vi "Main.vi"() -> ()   [LabVIEW 2014]
uses:
  <vilib>/myRIO/Common/Instrument Driver Framework/myRIO v1.0/PWM/vis/myRIO v1.1 Open PWM.vi
  <vilib>/myRIO/Common/Instrument Driver Framework/myRIO v1.0/UART/vis/myRIO v1.0 Close UART.vi
  <vilib>/myRIO/Common/Instrument Driver Framework/Utilities/vis/Validate Channels.vi
  <vilib>/myRIO/Common/Instrument Driver Framework/myRIO v1.0/PWM/vis/myRIO v1.0 Reserve PWM.vi
  <vilib>/myRIO/Common/Instrument Driver Framework/myRIO v1.0/PWM/vis/myRIO v1.0 Build MUX Configuration PWM.vi
  <vilib>/myRIO/Common/Instrument Driver Framework/myRIO v1.0/Resource Manager/vis/myRIO v1.0 Reserve Channel List.vi
  <vilib>/myRIO/Common/Instrument Driver Framework/myRIO v1.0/Resource Manager/vis/myRIO v1.0 Create Configuration List.vi
  <vilib>/myRIO/Common/Instrument Driver Framework/myRIO v1.0/Resource Manager/vis/myRIO v1.0 Reserve Channel.vi
  <vilib>/myRIO/Common/Instrument Driver Framework/myRIO v1.0/Resource Manager/vis/myRIO v1.0 Unreserve Channel.vi
  <vilib>/myRIO/Common/Instrument Driver Framework/myRIO v1.0/Resource Manager/vis/myRIO v1.0 Build Mutex Name.vi
  <vilib>/Utility/VariantDataType/GetNumericInfo.vi
  <vilib>/Utility/error.llb/Error Cluster From Error Code.vi
  <vilib>/myRIO/Common/Instrument Driver Framework/myRIO v1.0/myRIO v1.1 Open.vi
  <vilib>/myRIO/Common/Instrument Driver Framework/Utilities/vis/IO Manager.vi
  <vilib>/myRIO/Common/Instrument Driver Framework/Utilities/vis/Configuration Manager.vi
  <vilib>/myRIO/Common/Instrument Driver Framework/myRIO v1.0/Resource Manager/vis/myRIO v1.0 Configure IO.vi
  <vilib>/myRIO/Common/Instrument Driver Framework/myRIO v1.0/myRIO v1.0 Close.vi
  <vilib>/myRIO/Common/Instrument Driver Framework/myRIO v1.0/PWM/vis/myRIO v1.0 Write PWM.vi
  <vilib>/myRIO/Common/Instrument Driver Framework/Utilities/vis/FPGA Ref Manager.vi
  <vilib>/myRIO/Common/Instrument Driver Framework/myRIO v1.0/myRIO v1.0 Reset FPGA.vi
  <vilib>/myRIO/Common/Instrument Driver Framework/myRIO v1.0/IRQ/vis/myRIO v1.0 IRQ Info FGV.vi
  <vilib>/myRIO/Common/Instrument Driver Framework/myRIO v1.0/IRQ/vis/myRIO v1.0 Timer IRQ Info FGV.vi
  <vilib>/myRIO/Common/Instrument Driver Framework/myRIO v1.0/IRQ/vis/myRIO v1.0 ISR Agent.vi
  <vilib>/myRIO/Instrument Drivers/Utilities/Utilities.lvlib
  <vilib>/myRIO/Instrument Drivers/Onboard IO/PWM/PWM.lvlib
panel:
  in  "freq [Hz] 4":dbl=50.0
  in  "null offset 4":bool
  in  "position [%FS] 4":dbl(slide) scale=-200.0..200.0
  out "duty cycle [%] 4":dbl
  out "pulse width [ms] 4":dbl=1.5
  out "offset [%FS] 4":dbl
  out "pulse width [ms] 3":dbl=1.5
  out "duty cycle [%] 3":dbl
  out "offset [%FS] 3":dbl
  in  "null offset 3":bool
  in  "freq [Hz] 3":dbl=50.0
  in  "position [%FS] 3":dbl(slide) scale=-200.0..200.0
  in  "freq [Hz] 2":dbl=50.0
  in  "null offset 2":bool
  in  "position [%FS] 2":dbl(slide) scale=-200.0..200.0
  out "duty cycle [%] 2":dbl
  out "pulse width [ms] 2":dbl=1.5
  out "offset [%FS] 2":dbl
  out "duty cycle [%]":dbl
  out "pulse width [ms]":dbl=1.5
  out "offset [%FS]":dbl
  in  "freq [Hz]":dbl=50.0
  in  "null offset":bool
  in  "position [%FS]":dbl(slide) scale=-200.0..200.0
  in  "[ESC]":bool
  # "Servo  1"
  # "Servo  2"
  # "Servo  4"
  # "Servo  3"
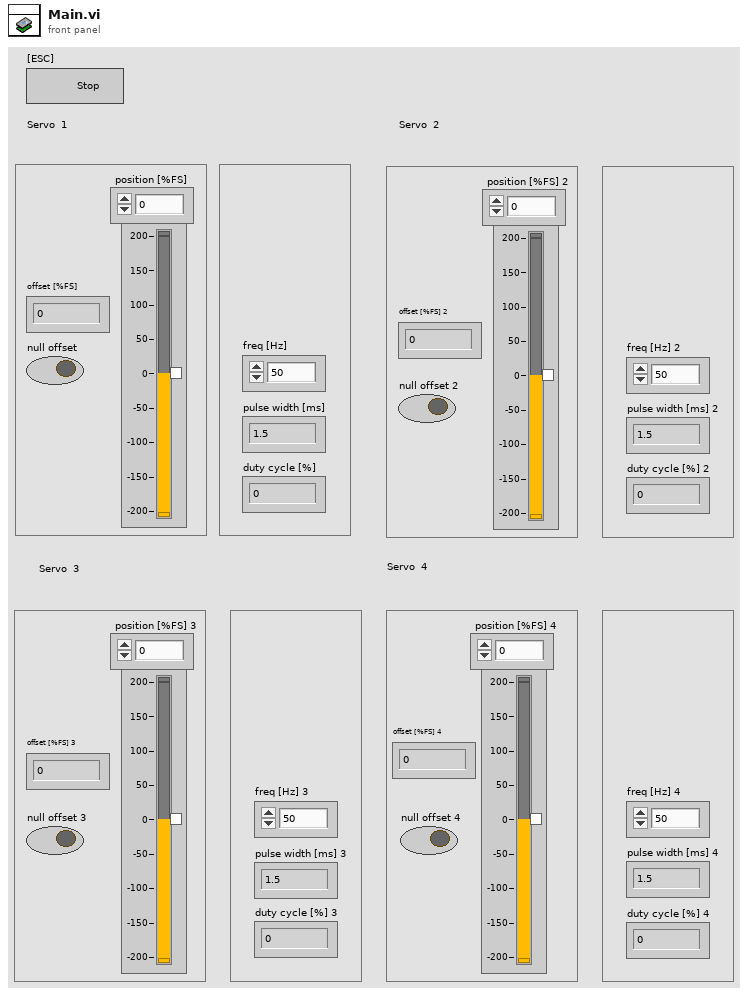
[diagram p1: front panel]
types:
  T1 = typedef "PWM.lvlib/PWM Reference.ctl" = cluster{"myRIO Reference":T2, "PWM Channels Enum":T6, "PWM Configuration":T7}
  T2 = typedef "myRIO Generic Hardware Reference.ctl" = cluster{"myRIO Model":T3, "myRIO Hardware Reference":T4}
  T3 = typedef "Hardware Version Enum.ctl" = enum16{"Unknown", "myRIO-1900", "myRIO-1950"}
  T4 = typedef "myRIO v1.0 Reference.ctl" = cluster{"Generic FPGA Reference":T5, "Allow multiple opens":bool}
  T5 = typedef "Generic FPGA Reference.ctl" = refnum<k20>
  T6 = typedef "PWM Channels Enum.ctl" = enum16{"Not Connected", "C/PWM0", "C/PWM1", "A/PWM0", "A/PWM1", "A/PWM2", "B/PWM0", "B/PWM1", "B/PWM2"}
  T7 = typedef "PWM.lvlib/PWM Configuration.ctl" = cluster{"Frequency":dbl, "Duty Cycle":dbl}
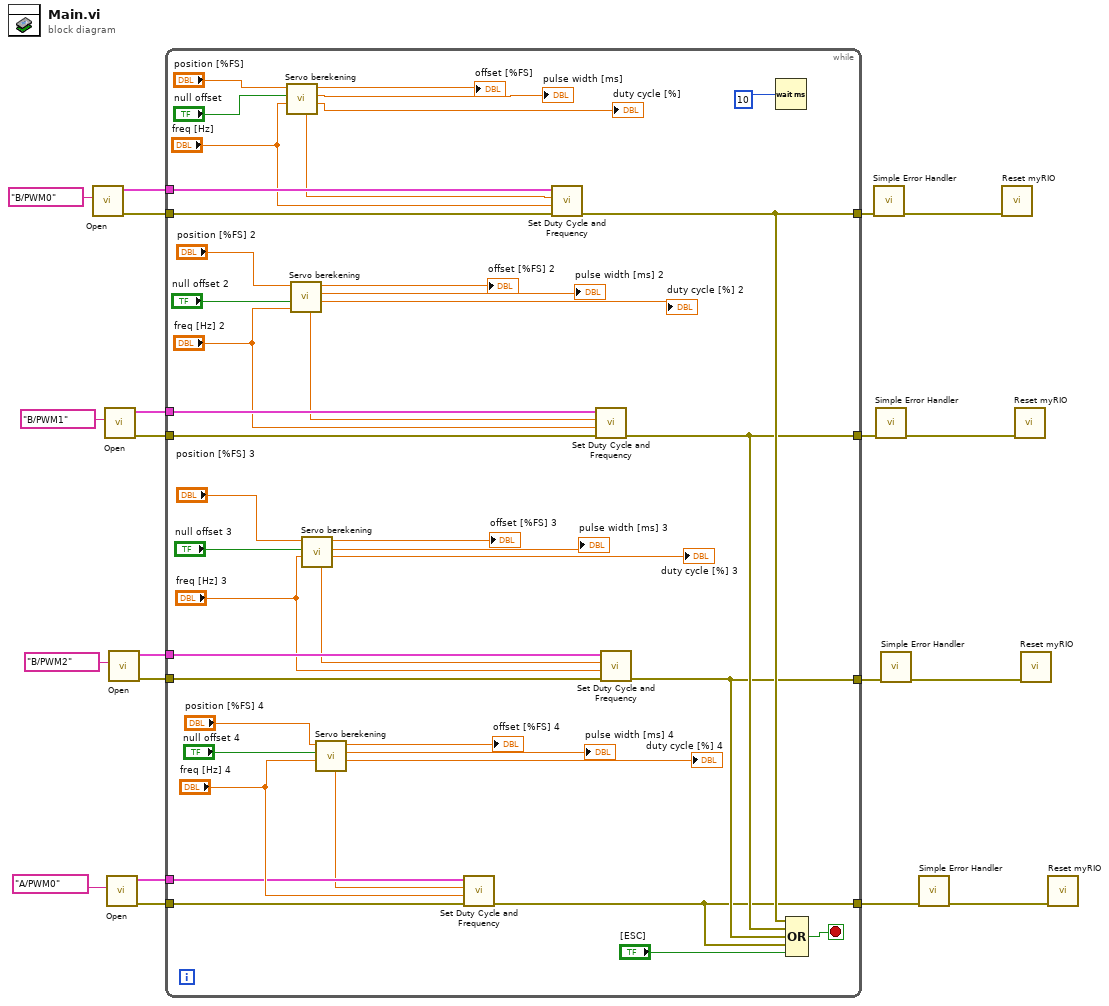
[diagram p0: block diagram]
diagram:
  n1 = call <vilib>:"Open.vi"("Channel Name"=tag "B/PWM0") -> ("error out"=w18:errorcluster, "PWM Ref Out"=w19:T1)  [unwired: 9 in]
  n2 = call <vilib>:"Open.vi"("Channel Name"=tag "B/PWM1") -> ("error out"=w15:errorcluster, "PWM Ref Out"=w14:T1)  [unwired: 9 in]
  n3 = call <vilib>:"Open.vi"("Channel Name"=tag "A/PWM0") -> ("error out"=w4:errorcluster, "PWM Ref Out"=w3:T1)  [unwired: 9 in]
  n4 = call <vilib>:"Open.vi"("Channel Name"=tag "B/PWM2") -> ("error out"=w13:errorcluster, "PWM Ref Out"=w12:T1)  [unwired: 9 in]
  n5 = while {
    tunnel: w19 -> [w62]
    tunnel: w18 -> [w61]
    tunnel: [w43] -> w17
    tunnel: w15 -> [w56]
    tunnel: w14 -> [w57]
    tunnel: w13 -> [w54]
    tunnel: w12 -> [w55]
    tunnel: [w42] -> w11
    tunnel: [w41] -> w10
    tunnel: w4 -> [w24]
    tunnel: w3 -> [w23]
    tunnel: [w22] -> w1
    stop <- w44 stop-if-true
    n6 = call "Servo berekening.vi"("freq [Hz]"="freq [Hz]", "null offset"="null offset", "position [%FS] in"="position [%FS]") -> ("Duty Cycle [%]"=→"duty cycle [%]":dbl, "Puls Width [ms]"=→"pulse width [ms]":dbl, "position [%FS] out"=→"offset [%FS]":dbl, "Duty Cycle"=w39:dbl)  [unwired: 5 in]
    n7 = call "Servo berekening.vi"("freq [Hz]"="freq [Hz] 2", "null offset"="null offset 2", "position [%FS] in"="position [%FS] 2") -> ("Duty Cycle [%]"=→"duty cycle [%] 2":dbl, "Puls Width [ms]"=→"pulse width [ms] 2":dbl, "position [%FS] out"=→"offset [%FS] 2":dbl, "Duty Cycle"=w38:dbl)  [unwired: 5 in]
    n8 = call "Servo berekening.vi"("freq [Hz]"="freq [Hz] 3", "null offset"="null offset 3", "position [%FS] in"="position [%FS] 3") -> ("Duty Cycle [%]"=→"duty cycle [%] 3":dbl, "Puls Width [ms]"=→"pulse width [ms] 3":dbl, "position [%FS] out"=→"offset [%FS] 3":dbl, "Duty Cycle"=w33:dbl)  [unwired: 5 in]
    n9 = call "Servo berekening.vi"("freq [Hz]"="freq [Hz] 4", "null offset"="null offset 4", "position [%FS] in"="position [%FS] 4") -> ("Duty Cycle [%]"=→"duty cycle [%] 4":dbl, "Puls Width [ms]"=→"pulse width [ms] 4":dbl, "position [%FS] out"=→"offset [%FS] 4":dbl, "Duty Cycle"=w21:dbl)  [unwired: 5 in]
    n10 = call <vilib>:"Set Duty Cycle and Frequency.vi"("error in (no error)"=w24, "Frequency [Hz]"="freq [Hz] 4", "Duty Cycle"=w21, "PWM Ref In"=w23) -> ("error out"=w22:errorcluster)  [unwired: 5 in, 1 out]
    n11 = call <vilib>:"Set Duty Cycle and Frequency.vi"("error in (no error)"=w61, "Frequency [Hz]"="freq [Hz]", "Duty Cycle"=w39, "PWM Ref In"=w62) -> ("error out"=w43:errorcluster)  [unwired: 5 in, 1 out]
    n12 = call <vilib>:"Set Duty Cycle and Frequency.vi"("error in (no error)"=w56, "Frequency [Hz]"="freq [Hz] 2", "Duty Cycle"=w38, "PWM Ref In"=w57) -> ("error out"=w42:errorcluster)  [unwired: 5 in, 1 out]
    n13 = call <vilib>:"Set Duty Cycle and Frequency.vi"("error in (no error)"=w54, "Frequency [Hz]"="freq [Hz] 3", "Duty Cycle"=w33, "PWM Ref In"=w55) -> ("error out"=w41:errorcluster)  [unwired: 5 in, 1 out]
    n14 = Wait (ms)(milliseconds to wait=u32 10) -> ()  [unwired: 1 out]
    n15 = Compound Arithmetic op=OR(w43, w42, w41, w22, "[ESC]") -> (w44:bool)
  }
  n16 = call <vilib>:"Simple Error Handler.vi"("error in (no error)"=w17) -> ("error out"=w20:errorcluster)  [unwired: 4 in, 4 out]
  n17 = call <vilib>:"Simple Error Handler.vi"("error in (no error)"=w11) -> ("error out"=w9:errorcluster)  [unwired: 4 in, 4 out]
  n18 = call <vilib>:"Simple Error Handler.vi"("error in (no error)"=w10) -> ("error out"=w8:errorcluster)  [unwired: 4 in, 4 out]
  n19 = call <vilib>:"Simple Error Handler.vi"("error in (no error)"=w1) -> ("error out"=w16:errorcluster)  [unwired: 4 in, 4 out]
  n20 = call <vilib>:"Reset myRIO.vi"("error in (no error)"=w20) -> ()  [unwired: 10 in, 1 out]
  n21 = call <vilib>:"Reset myRIO.vi"("error in (no error)"=w9) -> ()  [unwired: 10 in, 1 out]
  n22 = call <vilib>:"Reset myRIO.vi"("error in (no error)"=w8) -> ()  [unwired: 10 in, 1 out]
  n23 = call <vilib>:"Reset myRIO.vi"("error in (no error)"=w16) -> ()  [unwired: 10 in, 1 out]
